vi "Calcy.vi"() -> ()   [LabVIEW 2025]
panel:
  in  "CLR":bool
  out "String":string
  in  "Keypad":T1
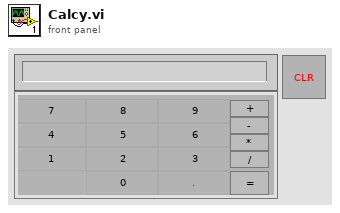
[diagram p1: front panel]
types:
  T1 = cluster{"0":bool, "1":bool, "2":bool, "3":bool, "4":bool, "5":bool, "6":bool, "7":bool, "8":bool, "9":bool, "decipoint":bool, "Add":bool, "Sub 3":bool, "Mul":bool, "Div":bool, "Equ":bool}
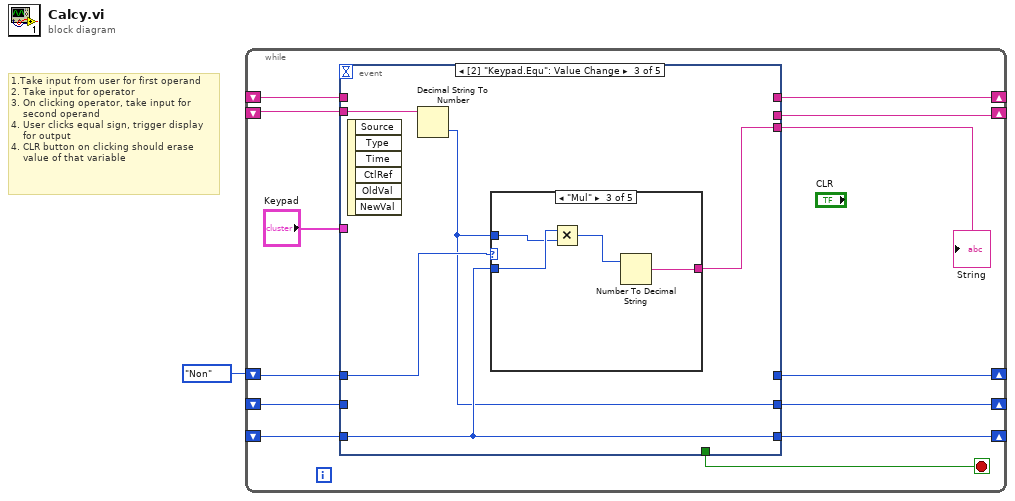
[diagram p0: block diagram]
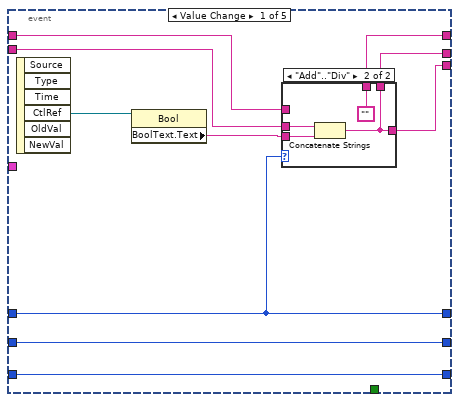
[diagram p2: hidden frame]
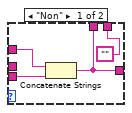
[diagram p3: hidden frame]
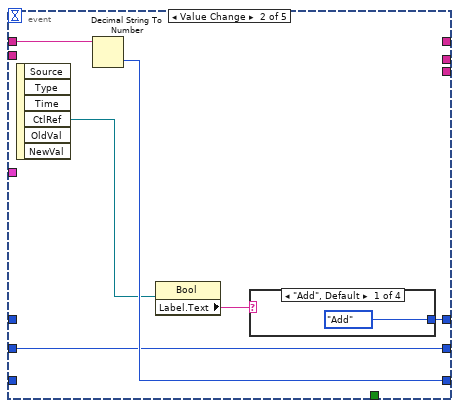
[diagram p4: hidden frame]
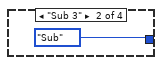
[diagram p5: hidden frame]
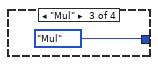
[diagram p6: hidden frame]
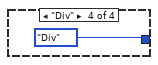
[diagram p7: hidden frame]
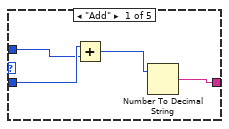
[diagram p8: hidden frame]
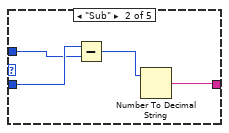
[diagram p9: hidden frame]
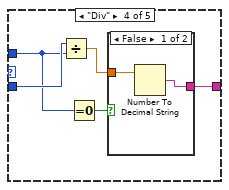
[diagram p10: hidden frame]
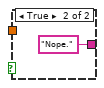
[diagram p11: hidden frame]
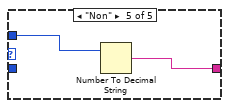
[diagram p12: hidden frame]
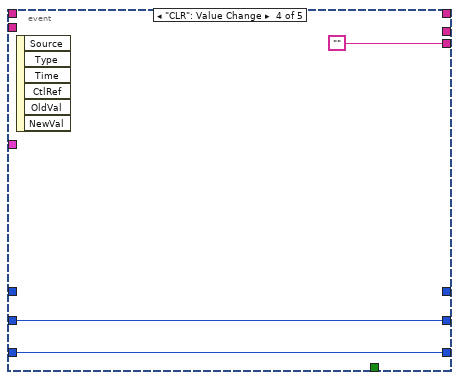
[diagram p13: hidden frame]
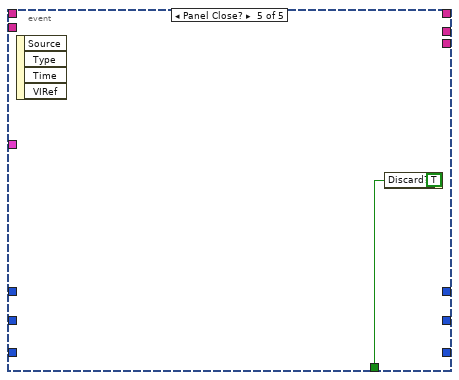
[diagram p14: hidden frame]
diagram:
  # "1.Take input from user for first operand\n2. Take input for operator\n3. On clicking operator, take input for\n    second operand\n4. User clicks equal sign, trigger display\n    for output\n4. CLR button on clicking should erase\n    value of that variable"
  n1 = while {
    shift-right: [w4] -> _
    shift-left: _ -> [w13]
    shift-right: [w12] -> _
    shift-left: _ -> [w11]
    shift-right: [w10] -> _
    shift-left: _ -> [w9]
    shift-right: [w7] -> _
    shift-left: enum16{"Add", "Sub", "Mul", "Div", "Non"}."Non" -> [w6]
    shift-right: [w3] -> _
    shift-left: _ -> [w5]
    stop <- w14 stop-if-true
    n2 = event shown="[2] \"Keypad.Equ\": Value Change" {
      selector: _ -> [_ _ _ _ _]
      dyn-events: _ -> [_ _ _ _ _]
      timeout: _ -> [_ _ _ _ _]
      tunnel: [_ _ _ _ w73] -> w14
      tunnel: [w18 _ w43 "" _] -> w8
      tunnel: w13 -> [w20 w38 _ _ _]
      tunnel: [w23 w37 w46 w71 _] -> w12
      tunnel: w11 -> [w23 _ w46 w71 _]
      tunnel: [w22 w33 w44 w70 _] -> w10
      tunnel: w9 -> [w22 w33 _ w70 _]
      tunnel: [w21 w35 _ _ _] -> w7
      tunnel: w6 -> [w21 _ w47 _ _]
      tunnel: w5 -> [w17 _ w45 _ _]
      tunnel: [w16 _ _ _ _] -> w4
      tunnel: [w15 _ _ _ _] -> w3
      tunnel: "Keypad" -> [_ _ _ _ _]
      event "Keypad.1", "Keypad.2", "Keypad.3", "Keypad.4", "Keypad.5", "Keypad.6", "Keypad.7", "Keypad.8", "Keypad.9", "Keypad.0": Value Change {
        n3 = event-data() -> ("CtlRef"=w24:refnum<vi>)  [unwired: 1 in, 5 out]
        n4 = property class="Bool"(reference=w24) -> ("BoolText.Text"=w19:string)  [unwired: 1 in, 2 out]
        n5 = case shown="\"Add\"..\"Div\"" w21 {
          tunnel: w20 -> [w28 _]
          tunnel: w19 -> [w27 w32]
          tunnel: [w26 w30] -> w18
          tunnel: w17 -> [_ w31]
          tunnel: [w26 ""] -> w16
          tunnel: ["" w30] -> w15
          frame "Non" {
            n6 = Concatenate Strings(w28, w27) -> (w26:string)
          }
          frame "Add".."Div" {
            n7 = Concatenate Strings(w31, w32) -> (w30:string)
          }
        }
      }
      event "Keypad.Add", "Keypad.Sub 3", "Keypad.Mul", "Keypad.Div": Value Change {
        n8 = event-data() -> ("CtlRef"=w36:refnum<vi>)  [unwired: 1 in, 5 out]
        n9 = Decimal String To Number(string=w38) -> (number=w37:i32)  [unwired: 2 in, 1 out]
        n10 = property on="Property Node" class="Bool"(reference=w36) -> ("Label.Text"=w34:string)  [unwired: 1 in, 2 out]
        n11 = case shown="\"Add\", Default" w34 {
          tunnel: [enum16{"Add", "Sub", "Mul", "Div", "Non"}."Add" enum16{"Add", "Sub", "Mul", "Div", "Non"}."Sub" enum16{"Add", "Sub", "Mul", "Div", "Non"}."Mul" enum16{"Add", "Sub", "Mul", "Div", "Non"}."Div"] -> w35
          frame "Add", Default {
          }
          frame "Sub 3" {
          }
          frame "Mul" {
          }
          frame "Div" {
          }
        }
      }
      event "Keypad.Equ": Value Change {
        n12 = event-data() -> ()  [unwired: 1 in, 6 out]
        n13 = Decimal String To Number(string=w45) -> (number=w44:i32)  [unwired: 2 in, 1 out]
        n14 = case shown="\"Mul\"" w47 {
          tunnel: w44 -> [w50 w54 w58 w63 w68]
          tunnel: w46 -> [w51 w55 w59 w64 _]
          tunnel: [w48 w53 w57 w61 w69] -> w43
          frame "Add" {
            n15 = Add(x=w51, y=w50) -> (x+y=w49:i32)
            n16 = Number To Decimal String(number=w49) -> (decimal integer string=w48:string)  [unwired: 1 in]
          }
          frame "Sub" {
            n17 = Subtract(x=w55, y=w54) -> (x-y=w52:i32)
            n18 = Number To Decimal String(number=w52) -> (decimal integer string=w53:string)  [unwired: 1 in]
          }
          frame "Mul" {
            n19 = Multiply(x=w59, y=w58) -> (x*y=w56:i32)
            n20 = Number To Decimal String(number=w56) -> (decimal integer string=w57:string)  [unwired: 1 in]
          }
          frame "Div" {
            n21 = Divide(x=w64, y=w63) -> (x/y=w60:dbl)
            n22 = Equal To 0?(x=w63) -> (x = 0?=w62:bool)
            n23 = case shown="False" w62 {
              tunnel: [w66 "Nope."] -> w61
              tunnel: w60 -> [w65 _]
              frame False {
                n24 = Number To Decimal String(number=w65) -> (decimal integer string=w66:string)  [unwired: 1 in]
              }
              frame True {
              }
            }
          }
          frame "Non" {
            n25 = Number To Decimal String(number=w68) -> (decimal integer string=w69:string)  [unwired: 1 in]
          }
        }
      }
      event "CLR": Value Change {
        n26 = event-data() -> ()  [unwired: 1 in, 6 out]
      }
      event Panel Close? {
        w73 = TRUE ("Discard?")
        n27 = event-data() -> ()  [unwired: 1 in, 4 out]
        n28 = event-data("Discard?"=w73) -> ()  [unwired: 1 in, 1 out]
      }
    }
    "String" <- w8
  }
